vi "Set Wait.vi"(6 "Write to FPGA(T)":bool=TRUE, 8 "error in (no error)":errorcluster, 10 "Duration":u32, 11 "FPGA VI Reference In":refnum<k20>) -> (0 "error out":errorcluster, 3 "FPGA VI Reference Out":refnum<k20>)   [LabVIEW 2016]
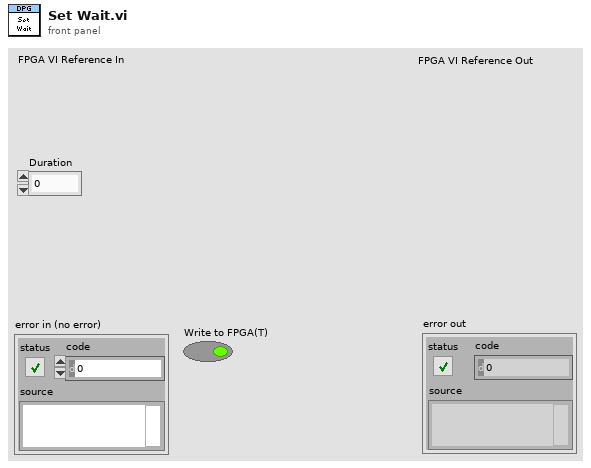
[diagram p1: front panel]
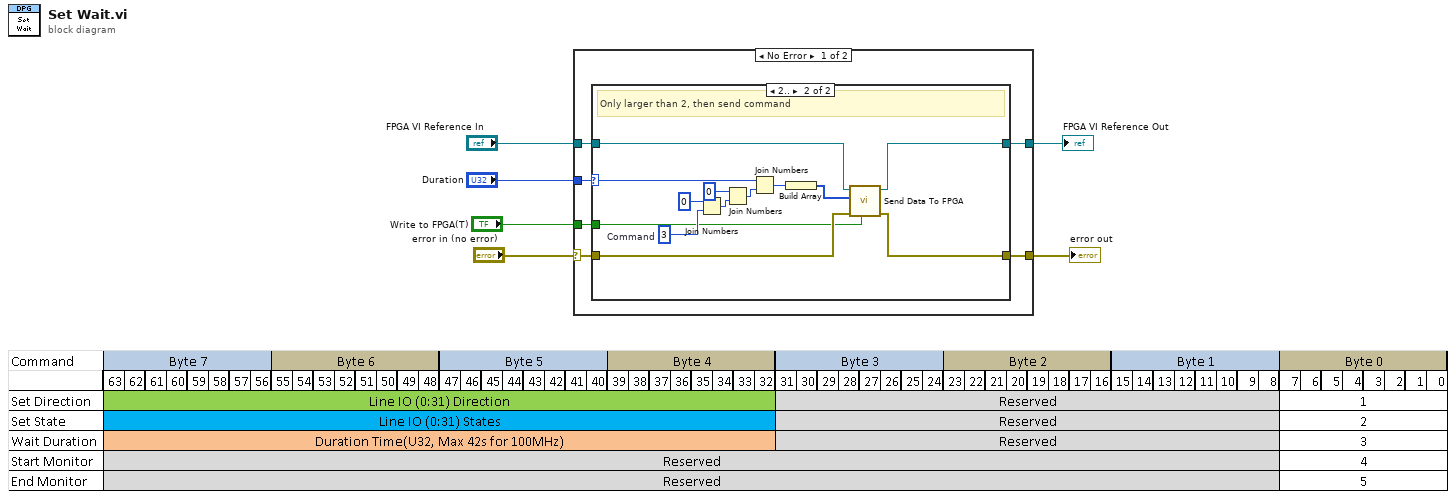
[diagram p0: block diagram]
diagram:
  n1 = case shown="No Error" "error in (no error)" {
    selector: "error in (no error)" -> [w11 w29]
    tunnel: "FPGA VI Reference In" -> [w12 w28]
    tunnel: [w9 w29] -> w4
    tunnel: "Duration" -> [w8 _]
    tunnel: "Write to FPGA(T)" -> [w10 _]
    tunnel: [w7 w28] -> w1
    frame No Error {
      n2 = case shown="2.." w8 {
        selector: w8 -> [_ w16]
        tunnel: w12 -> [w13 w22]
        tunnel: w11 -> [w14 w19]
        tunnel: w10 -> [_ w18]
        tunnel: [w14 w17] -> w9
        tunnel: [w13 w15] -> w7
        frame 0, 1, Default {
          # "Set State takes 1 tick itself"
          # "No send command for less than 2"
        }
        frame 2.. {
          w25 = u16 3  # Command
          # "Only larger than 2, then send command"
          n3 = Join Numbers(hi=u16 0, lo=w25) -> ((hi.lo)=w26:u32)
          n4 = Join Numbers(hi=u32 0, lo=w26) -> ((hi.lo)=w27:u64)
          n5 = Join Numbers(hi=w16, lo=w27) -> ((hi.lo)=w21:u64)
          n6 = Build Array(w21) -> (w20:u64[])
          n7 = call "Send Data To FPGA.vi"("Write to FPGA(T)"=w18, "error in (no error)"=w19, "Data"=w20, "FPGA VI Reference In"=w22) -> ("error out"=w17:errorcluster, "FPGA VI Reference Out"=w15:refnum<k20>)  [unwired: 6 in]
        }
      }
    }
    frame Error {
    }
  }
  "error out" <- w4
  "FPGA VI Reference Out" <- w1
